vi "Determine Properties Listbox Values.vi"(8 "error in (no error)":errorcluster, 10 "all properties":T1[](array[typedef]), 11 "Section Ref in":T2 format="%.0x") -> (0 "error out":errorcluster, 1 "not present item indexes":i32[](array[numeric]), 2 "listbox text":string[][](array[string]), 3 "Section Ref out":T2 format="%.0x")   [LabVIEW 2017]
uses:
  <vilib>/NI Veristand/Custom Device API/Custom Device Item Ref.ctl
  SLSC EDS API/JSON parsing/property.ctl
  <vilib>/NI Veristand/Custom Device API/Custom Device API.lvlib
  <vilib>/NI Veristand/Custom Device API/Get Item Property (String).vi
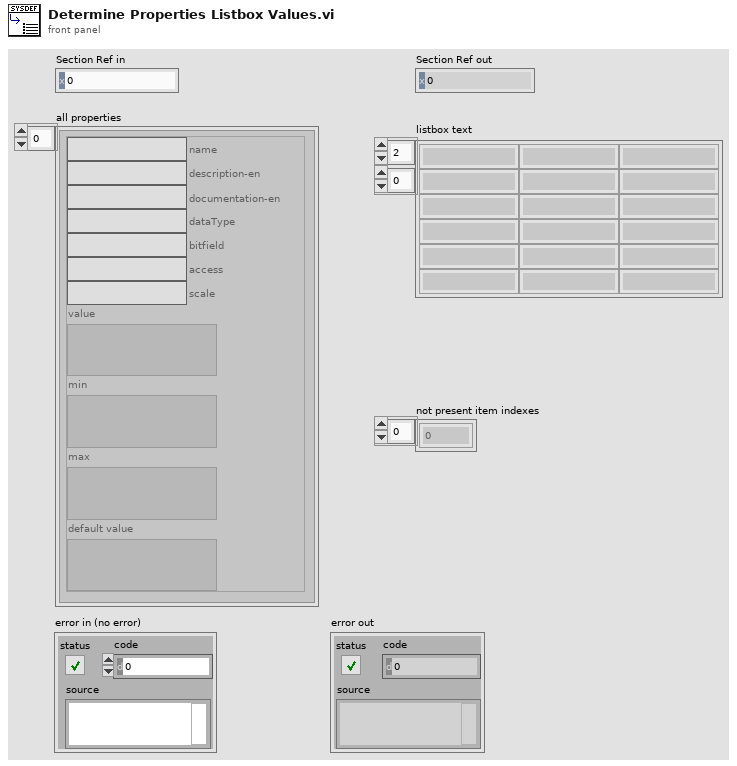
[diagram p1: front panel]
types:
  T1 = typedef "property.ctl" = cluster{"name":string, "description-en":string, "documentation-en":string, "dataType":string, "bitfield":string, "access":string, "scale":string, "value":variant, "min":variant, "max":variant, "default value":variant}
  T2 = typedef "Custom Device API.lvlib/Custom Device Item Ref.ctl" = u64
  T3 = typedef "Custom Device API.lvlib/Custom Device Item Info.ctl" = cluster{"Name":string, "Is Channel":bool, "GUID":string, "Is Waveform":bool}
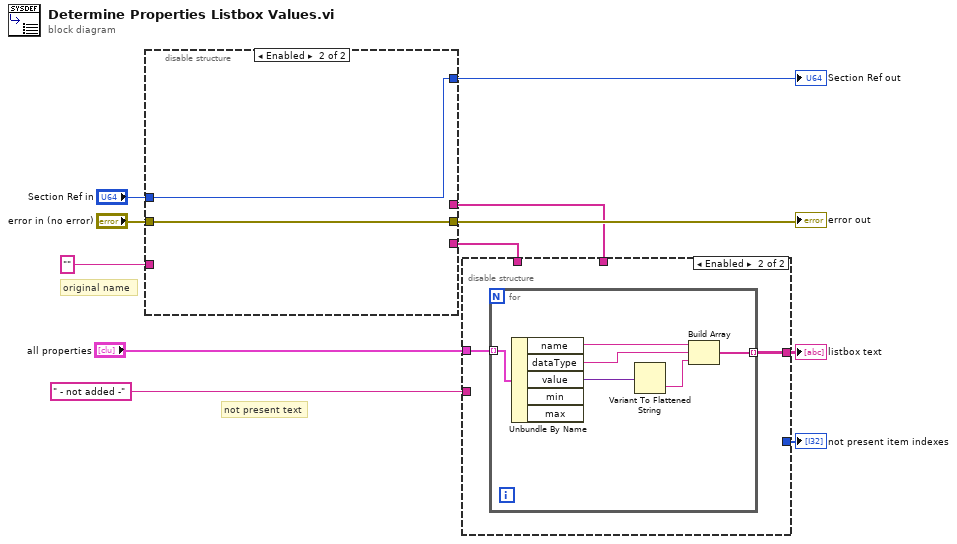
[diagram p0: block diagram]
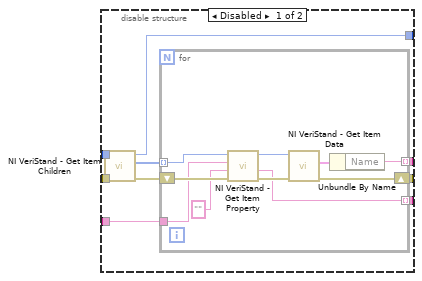
[diagram p2: hidden frame]
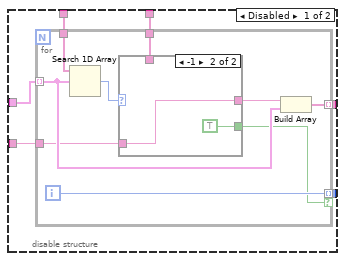
[diagram p3: hidden frame]
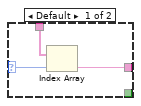
[diagram p4: hidden frame]
diagram:
  # "not present text"
  # "original name"
  n1 = disable-structure shown="Enabled" {
    disable-tunnel: "error in (no error)" -> [w20 w32]
    disable-tunnel: "Section Ref in" -> [w19 w31]
    disable-tunnel: [w16 w31] -> w9
    disable-tunnel: [w15 w32] -> w8
    disable-tunnel: [w14 _] -> w7
    disable-tunnel: [w13 _] -> w6
    disable-tunnel: "" -> [w12 _]
    frame Disabled {
      n2 = call <vilib>:"NI VeriStand - Get Item Children.vi"("error in (no error)"=w20, "Item Ref in"=w19) -> ("error out"=w18:errorcluster, "Child Refs"=w17:T2[], "Item Ref out"=w16:T2)  [unwired: 6 in, 1 out]
      n3 = for {
        shift-right: [w25] -> w15
        shift-left: w18 -> [w30]
        tunnel: w17 -> [w28] mode=indexing
        tunnel: w12 -> [w27]
        tunnel: [w22] -> w14 mode=indexing
        tunnel: [w21] -> w13 mode=indexing
        n4 = call-poly <vilib>:"NI VeriStand - Get Item Property.vi"("error in (no error)"=w30, "Default Value"="", "Property Name"=w27, "Item Ref in"=w28) -> ("error out"=w29:errorcluster, "Value"=w22:string, "Item Ref out"=w24:T2)  [unwired: 4 in, 1 out]
        n5 = call <vilib>:"NI VeriStand - Get Item Data.vi"("error in (no error)"=w29, "Item Ref in"=w24) -> ("error out"=w25:errorcluster, "Item Info"=w23:T3)  [unwired: 6 in, 2 out]
        n6 = Unbundle By Name(w23) -> ("Name"=w21:string)
      }
    }
    frame Enabled {
    }
  }
  "error out" <- w8
  "Section Ref out" <- w9
  n7 = disable-structure shown="Enabled" {
    disable-tunnel: w7 -> [w38 _]
    disable-tunnel: w6 -> [w37 _]
    disable-tunnel: [w36 w53] -> w5
    disable-tunnel: [w35 _] -> w4
    disable-tunnel: " - not added -" -> [w34 _]
    disable-tunnel: "all properties" -> [w33 w54]
    frame Disabled {
      n8 = for {
        tunnel: w33 -> [w43] mode=indexing
        tunnel: w38 -> [w47]
        tunnel: w37 -> [w45]
        tunnel: [w42] -> w36 mode=indexing
        tunnel: w34 -> [w41]
        tunnel: [w40] -> w35 mode=indexing if=w39
        i -> [w40]
        n9 = Search 1D Array(1D array=w47, element=w43) -> (index of element=w46:i32)  [unwired: 1 in]
        n10 = case shown="-1" w46 {
          selector: w46 -> [w49 _]
          tunnel: [w48 w52] -> w44
          tunnel: w45 -> [w50 _]
          tunnel: w41 -> [_ w52]
          tunnel: [_ TRUE] -> w39
          frame Default {
            n11 = Index Array(array=w50, index=w49) -> (element=w48:string)
          }
          frame -1 {
          }
        }
        n12 = Build Array(w44, w43) -> (w42:string[])
      }
    }
    frame Enabled {
      n13 = for {
        tunnel: w54 -> [w60] mode=indexing
        tunnel: [w55] -> w53 mode=indexing
        n14 = Unbundle By Name(w60) -> ("name"=w58:string, "dataType"=w57:string, "value"=w59:variant)  [unwired: 2 out]
        n15 = Variant To Flattened String(Variant=w59) -> (data string=w56:string)  [unwired: 1 out]
        n16 = Build Array(w58, w57, w56) -> (w55:string[])
      }
    }
  }
  "listbox text" <- w5
  "not present item indexes" <- w4
